vi "SA_SET_REFSRC.vi"(0 "Session In":refnum<visa-resource-name>="TCPIP0::169.254.70.120::inst0::INSTR", 1 "Delay  (ms)":i64=1 caption="Delay Time (s)", 11 "error in":errorcluster {"code" format="%.0x"}, 12 "READ ONLY (T)":bool, 13 "REF_SRC [INT|EXT]":i32(ring) items=["INTERNAL", "EXTERNAL", "SENSE(XA Series)", "PULS(XA Series)"], 14 "Send OPC? (T)":bool=TRUE) -> (4 "Session Out":refnum<visa-resource-name>="TCPIP0::169.254.70.120::inst0::INSTR", 6 "READ":string="INT", 15 "error out":errorcluster {"code" format="%.0x"})   [LabVIEW 2018]
uses:
  Initialize References/Station References Global.vi
  Keysight N9010A/Agilent MXA Series/Agilent MXA Series.lvlib
panel:
  out "RD(CMD)":string="ROSC:SOUR?"
  out "WR(CMD)":string="SENS:ROSC:SOUR INT"
  out "IsPSA?(t)":bool=TRUE
  in  "Timeout":u32=3000
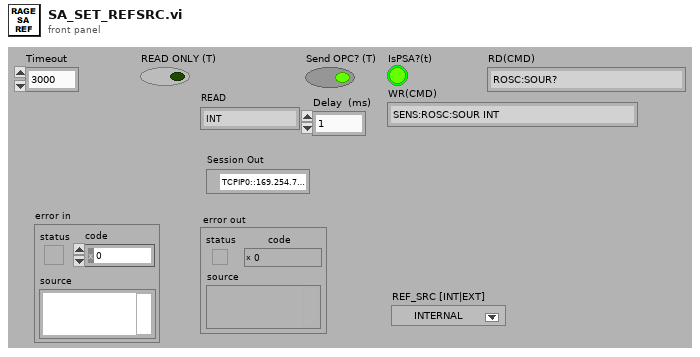
[diagram p1: front panel]
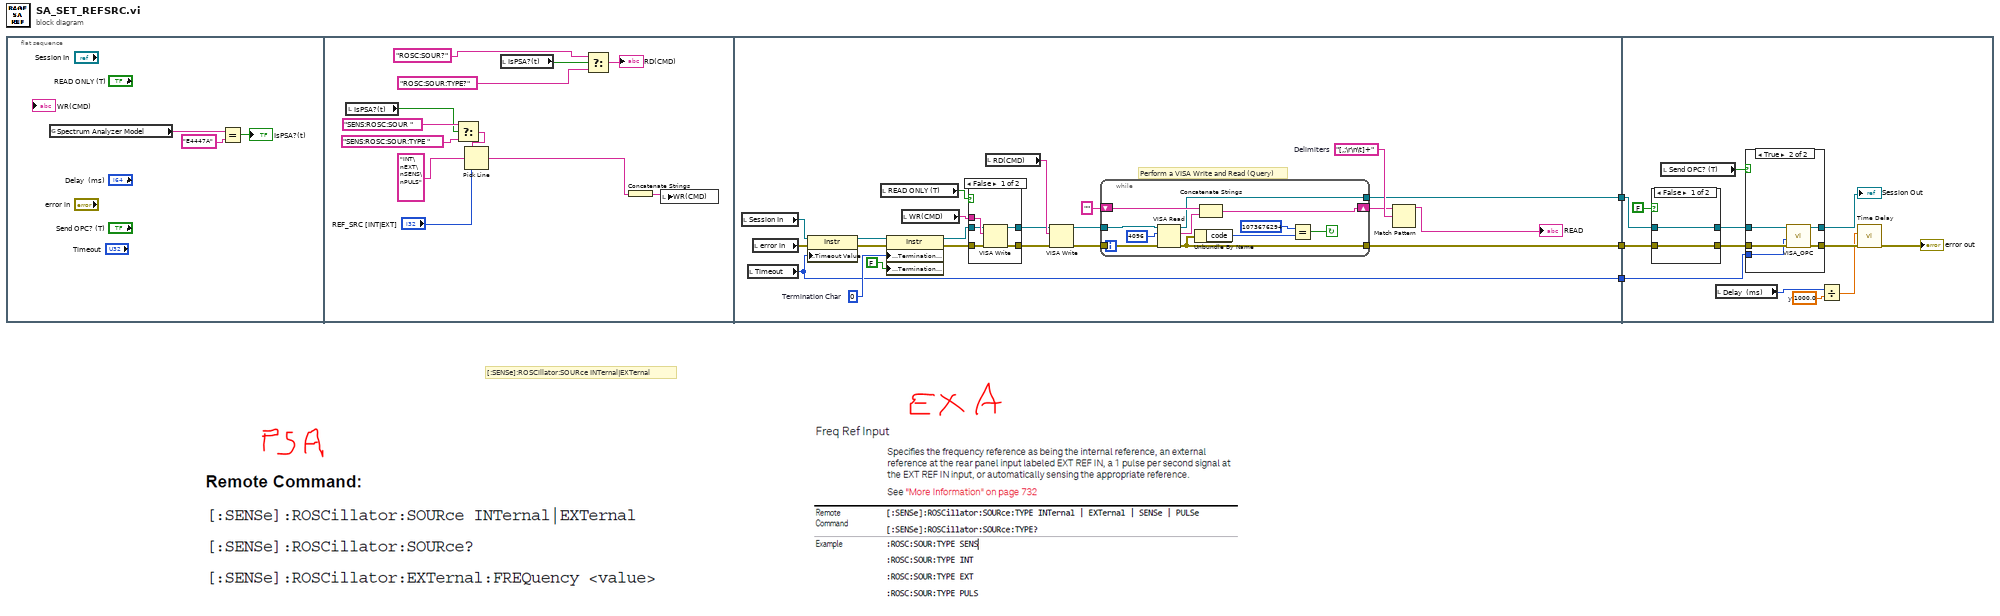
[diagram p0: block diagram]
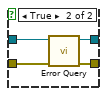
[diagram p4: hidden frame]
diagram:
  # "[:SENSe]:ROSCillator:SOURce INTernal|EXTernal"
  n1 = flat-sequence {
    tunnel: [w23] -> w3
    tunnel: [w22] -> w2
    tunnel: [w21] -> w1
    tunnel: w3 -> [w62]
    tunnel: w2 -> [w60]
    tunnel: w1 -> [w59]
    frame #0 {
      n2 = global read "Station References Global.vi" "Spectrum Analyzer Model"() -> (w6:string)
      n3 = Equal?(x=w6, y="E4447A") -> (x = y?=→"IsPSA?(t)":bool)
    }
    frame #1 {
      n4 = local read "IsPSA?(t)"() -> (w9:bool)
      n5 = Select(t="SENS:ROSC:SOUR " ("staticText"), s=w9, f="SENS:ROSC:SOUR:TYPE " ("staticText")) -> (s? t:f=w10:string)
      n6 = Pick Line(string ("")=w10, multi-line string="INT\nEXT\nSENS\nPULS", line index="REF_SRC [INT|EXT]") -> (output string=w8:string)
      n7 = local read "IsPSA?(t)"() -> (w15:bool)
      n8 = Select(t="ROSC:SOUR?", s=w15, f="ROSC:SOUR:TYPE?") -> (s? t:f=→"RD(CMD)":string)
      n9 = Concatenate Strings(w8) -> (w18:string)
      n10 = local write "WR(CMD)"(w18) -> ()
    }
    frame #2 {
      w27 = "[,;\r\n\t]+"  # Delimiters
      w25 = u8 0  # Termination Char
      # "Perform a VISA Write and Read (Query)"
      n11 = local read "Session In"() -> (w36:refnum<visa-resource-name>)
      n12 = local read "Timeout"() -> (w23:u32)
      n13 = local read "error in"() -> (w38:errorcluster)
      n14 = property class="Instr"(reference=w36, error in=w38, "General Settings:Timeout Value"=w23) -> (reference out=w30:refnum<visa-resource-name>, error out=w28:errorcluster)
      n15 = local read "READ ONLY (T)"() -> (w37:bool)
      n16 = property class="Instr"(reference=w30, error in=w28, "Message Based Settings:Termination Character"=w25, "Message Based Settings:Termination Character Enable"=FALSE ("enable")) -> (reference out=w34:refnum<visa-resource-name>, error out=w29:errorcluster)
      n17 = local read "WR(CMD)"() -> (w39:string)
      n18 = case shown="False" w37 {
        tunnel: w29 -> [w45 w46]
        tunnel: [w44 w46] -> w31
        tunnel: w39 -> [w43 _]
        tunnel: w34 -> [w42 w47]
        tunnel: [w41 w47] -> w35
        frame False {
          n19 = VISA Write(VISA resource name=w42, write buffer=w43, error in (no error)=w45) -> (VISA resource name out=w41:refnum<visa-resource-name>, error out=w44:errorcluster)  [unwired: 1 out]
        }
        frame True {
        }
      }
      n20 = local read "RD(CMD)"() -> (w40:string)
      n21 = VISA Write(VISA resource name=w35, write buffer=w40, error in (no error)=w31) -> (VISA resource name out=w32:refnum<visa-resource-name>, error out=w33:errorcluster)  [unwired: 1 out]
      n22 = while {
        tunnel: w32 -> [w55]
        shift-right: [w49] -> w20
        shift-left: "" -> [w54]
        tunnel: w33 -> [w52]
        tunnel: [w51] -> w21
        tunnel: [w48] -> w22
        stop <- w50 continue-if-true
        n23 = VISA Read(VISA resource name=w55, byte count=u32 4096 ("byte count (0)"), error in (no error)=w52) -> (VISA resource name out=w48:refnum<visa-resource-name>, read buffer=w53:string, error out=w51:errorcluster)  [unwired: 1 out]
        n24 = Unbundle By Name(w51) -> ("code"=w57:i32)
        n25 = Concatenate Strings(w54, w53) -> (w49:string)
        n26 = Equal?(x=1073676294, y=w57) -> (x = y?=w50:bool)
      }
      n27 = Match Pattern(string=w20, regular expression=w27) -> (before substring=→"READ":string)  [unwired: 4 out]
    }
    frame #3 {
      w63 = 1000.0  # y
      n28 = case shown="False" FALSE {
        tunnel: w60 -> [w79 w84]
        tunnel: [w79 w83] -> w70
        tunnel: w59 -> [w80 w82]
        tunnel: [w80 w81] -> w71
        frame False {
        }
        frame True {
          n29 = call "Error Query.vi"("error in (no error)"=w82, "VISA resource name"=w84) -> ("error out"=w81:errorcluster, "VISA resource name out"=w83:refnum<visa-resource-name>)  [unwired: 6 in, 2 out]
        }
      }
      n30 = local read "Send OPC? (T)"() -> (w64:bool)
      n31 = local read "Delay  (ms)"() -> (w65:i64)
      n32 = case shown="True" w64 {
        tunnel: w71 -> [w72 w78]
        tunnel: w70 -> [w73 w77]
        tunnel: [w73 w76] -> w69
        tunnel: [w72 w75] -> w68
        tunnel: w62 -> [_ w74]
        frame False {
        }
        frame True {
          n33 = call "VISA_OPC.vi"("error in"=w78, "Timeout"=w74, "Session In"=w77) -> ("error out"=w75:errorcluster, "Session Out"=w76:refnum<visa-resource-name>)  [unwired: 6 in, 1 out]
        }
      }
      "Session Out" <- w69
      n34 = Divide(x=w65, y=w63) -> (x/y=w66:dbl)
      n35 = call "Time Delay"("error in (no error)"=w68, "Delay Time (s)"=w66) -> ("error out"=→"error out":errorcluster)  [unwired: 9 in]
    }
  }
